vi "Write All Control Values.vi"(8 "error in (no error)":errorcluster, 11 "CD Parameter Manager in":refnum<class "CD Parameter Manager.lvclass">) -> (0 "error out":errorcluster, 3 "CD Parameter Manager out":refnum<class "CD Parameter Manager.lvclass">)   [LabVIEW 2019, in "CD Parameter Manager API.lvlib" / "CD Parameter Manager.lvclass"]
uses:
  CD Parameter Manager.lvclass
  CD Parameter Manager.lvclass/CD Parameter Manager.ctl
  Parameter Class/Parameter.lvclass
panel:
  in  "VI Ref":refnum<vi>
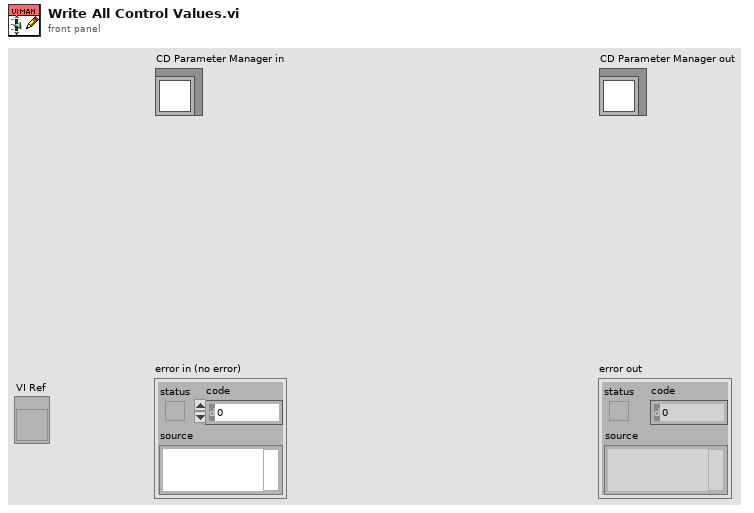
[diagram p1: front panel]
types:
  T1 = cluster{"Group name":string, "Controls":refnum<class "Parameter.lvclass">[]}[]
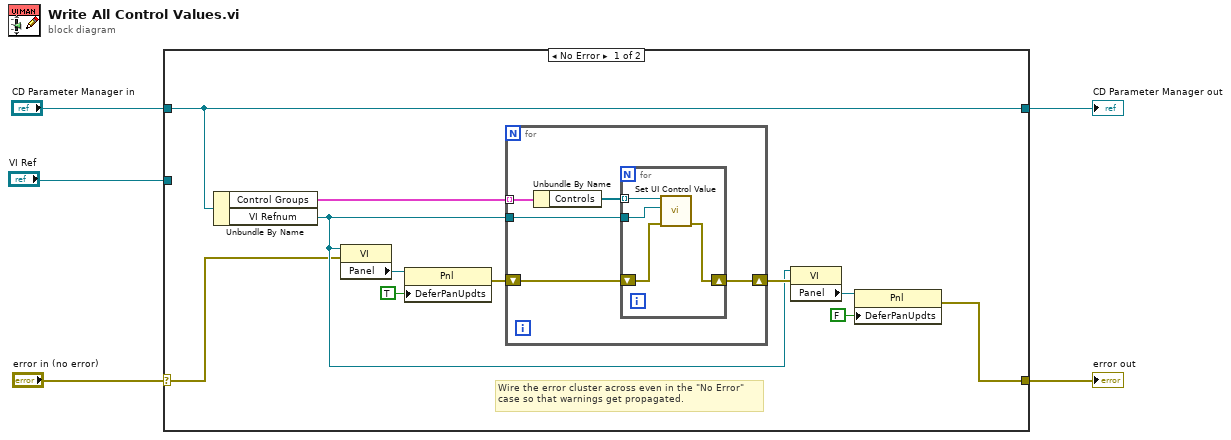
[diagram p0: block diagram]
diagram:
  n1 = case shown="No Error" "error in (no error)" {
    selector: "error in (no error)" -> [w6 w27]
    tunnel: [w8 w27] -> w4
    tunnel: [w16 w26] -> w2
    tunnel: "CD Parameter Manager in" -> [w16 w26]
    tunnel: "VI Ref" -> [_ _]
    frame No Error {
      # "Wire the error cluster across even in the \"No Error\"\ncase so that warnings get propagated."
      n2 = Unbundle By Name(w16) -> ("Control Groups"=w15:T1, "VI Refnum"=w7:refnum<vi>)
      n3 = property class="VI"(reference=w7, error in=w6) -> ("Panel"=w13:refnum<vi>)  [unwired: 2 out]
      n4 = property class="Pnl"(reference=w13, "DeferPanUpdts"=TRUE ("Defer Panel Updates")) -> (error out=w12:errorcluster)  [unwired: 1 in, 1 out]
      n5 = for {
        tunnel: w7 -> [w21]
        tunnel: w15 -> [w18] mode=indexing
        shift-right: [w19] -> w9
        shift-left: w12 -> [w20]
        n6 = Unbundle By Name(w18) -> ("Controls"=w17:refnum<class "Parameter.lvclass">[])
        n7 = for {
          tunnel: w21 -> [w25]
          shift-right: [w23] -> w19
          shift-left: w20 -> [w24]
          tunnel: w17 -> [w22] mode=indexing
          n8 = call-dynamic "Set UI Control Value.vi"("error in (no error)"=w24, "VI Ref"=w25, "Parameter in"=w22) -> ("error out"=w23:errorcluster)  [unwired: 7 in, 1 out]
        }
      }
      n9 = property class="VI"(reference=w7, error in=w9) -> ("Panel"=w11:refnum<vi>)  [unwired: 2 out]
      n10 = property class="Pnl"(reference=w11, "DeferPanUpdts"=FALSE ("Defer Panel Updates")) -> (error out=w8:errorcluster)  [unwired: 1 in, 1 out]
    }
    frame Error {
    }
  }
  "error out" <- w4
  "CD Parameter Manager out" <- w2
